vi "SCMP - Write Comments to File.vi"(8 "error in":errorcluster, 9 "data to end":string, 10 "data":string, 11 "Today's SCMP folder":path) -> (0 "error out":errorcluster, 2 "Last Log Entry":string="\r", 3 "Entire Log File":string="\n", 5 "Today's SCMP Log File":path)   [LabVIEW 2014]
doc: "This vi create or open file, which is save in format YYYYMMDD.txt. In this file are logs from CoMP-S Main program."
panel:
  in  "SCMP Log File":path=path "SCMP dump init.log"
  out "first call":bool
  out "date/time string":string="20141030"
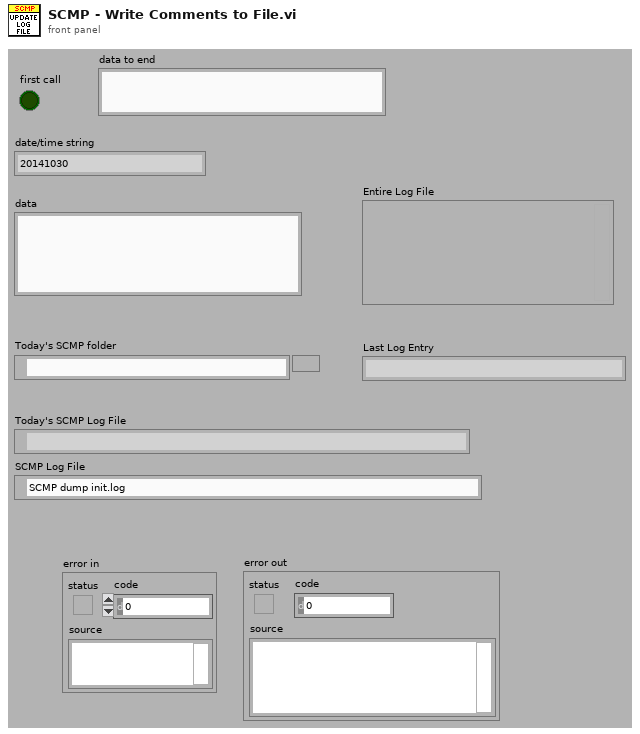
[diagram p1: front panel]
types:
  T1 = enum16{"open", "replace", "create", "open or create", "replace or create", "replace or create with confirmation"}
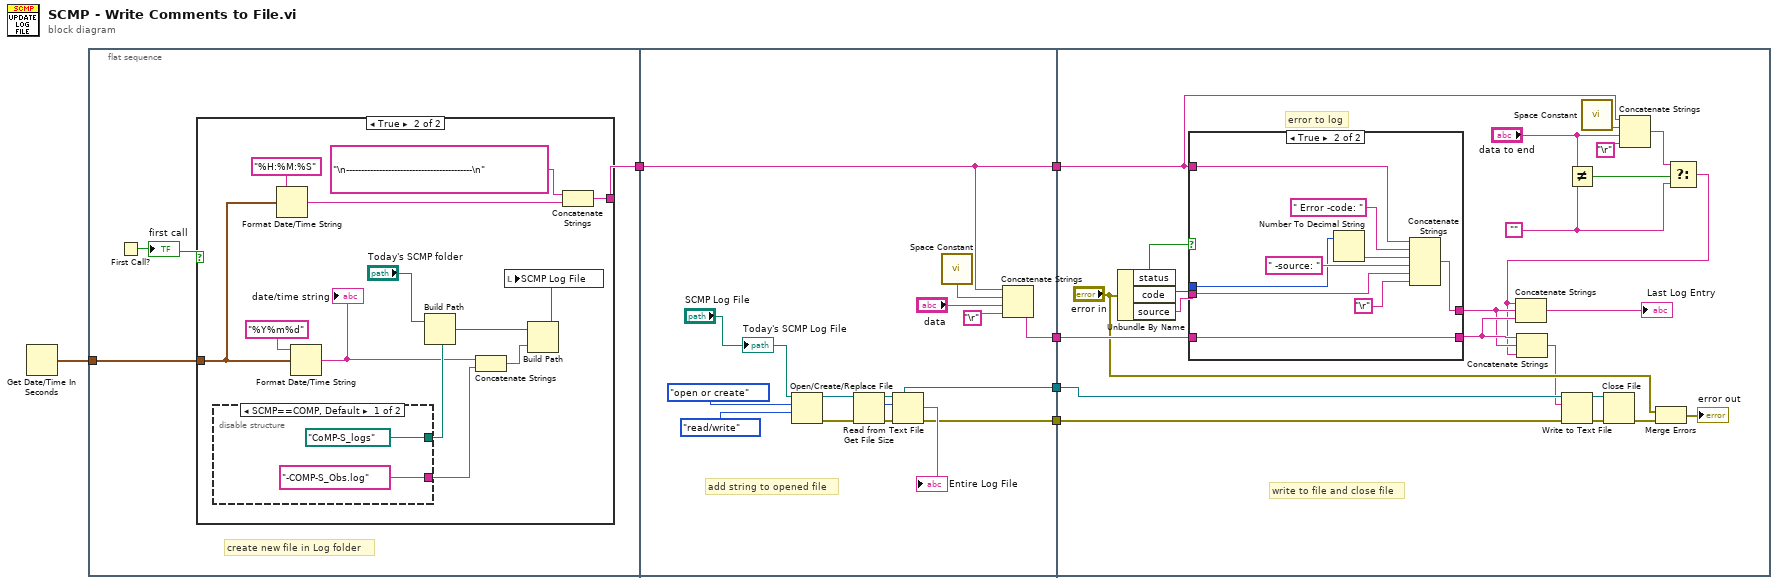
[diagram p0: block diagram]
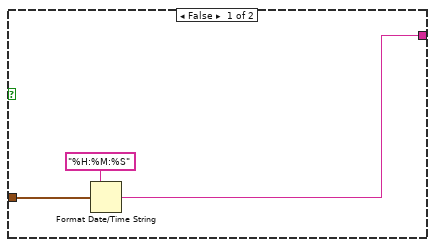
[diagram p2: hidden frame]
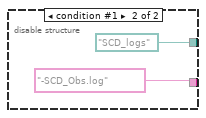
[diagram p3: hidden frame]
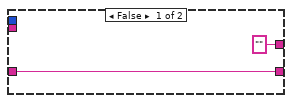
[diagram p4: hidden frame]
diagram:
  n1 = Get Date/Time In Seconds() -> (seconds since 1Jan1904=w3:timestamp)
  n2 = flat-sequence {
    tunnel: w3 -> [w8]
    tunnel: [w7] -> w1
    tunnel: [w34] -> w6
    tunnel: [w35] -> w5
    tunnel: [w30] -> w4
    tunnel: [w32] -> w2
    tunnel: w1 -> [w30]
    tunnel: w6 -> [w62]
    tunnel: w5 -> [w66]
    tunnel: w4 -> [w47]
    tunnel: w2 -> [w61]
    frame #0 {
      # "create new file in Log folder"
      n3 = First Call?() -> (First Call?: T/F=w9:bool)
      "first call" <- w9
      n4 = case shown="True" w9 {
        tunnel: w8 -> [w11 w16]
        tunnel: [w10 w14] -> w7
        frame False {
          n5 = Format Date/Time String(time format string (%c)="%H:%M:%S", seconds (now)=w11) -> (date/time string=w10:string)  [unwired: 1 in]
        }
        frame True {
          n6 = disable-structure shown="SCMP==COMP, Default" {
            disable-tunnel: [path "CoMP-S_logs" path "SCD_logs"] -> w24
            disable-tunnel: ["-COMP-S_Obs.log" ("string") "-SCD_Obs.log" ("string")] -> w20
            frame condition #0 (active) {
            }
            frame condition #1 {
            }
          }
          n7 = Format Date/Time String(time format string (%c)="%H:%M:%S", seconds (now)=w16) -> (date/time string=w13:string)  [unwired: 1 in]
          n8 = Format Date/Time String(time format string (%c)="%Y%m%d", seconds (now)=w16) -> (date/time string=w21:string)  [unwired: 1 in]
          "date/time string" <- w21
          n9 = Build Path(base path="Today's SCMP folder", name or relative path=w24) -> (appended path=w23:path)
          n10 = Concatenate Strings(w21, w20) -> (w22:string)
          n11 = Build Path(base path=w23, name or relative path=w22) -> (appended path=w19:path)
          n12 = local write "SCMP Log File"(w19) -> ()
          n13 = Concatenate Strings("\n------------------------------------------\n" ("date/time string"), w13) -> (w14:string)
        }
      }
    }
    frame #1 {
      # "add string to opened file"
      n14 = Open/Create/Replace File(file path (use dialog)="SCMP Log File", operation (0:open)=T1."open or create", access (0:read/write)=enum16{"read/write", "read-only", "write-only"}."read/write") -> (refnum out=w42:refnum<file>, error out=w41:errorcluster)  [unwired: 1 in, 3 out]
      n15 = Get File Size(file=w42, error in=w41) -> (refnum out=w43:refnum<file>, size (in bytes)=w44:i64, 0:w33:errorcluster)
      n16 = Read from Text File(file (use dialog)=w43, count=w44, error in=w33) -> (refnum out=w35:refnum<file>, text=→"Entire Log File":string, error out=w32:errorcluster)  [unwired: 2 out]
      n17 = call <vilib>:"Space Constant.vi"() -> ("String"=w39:string)
      n18 = Concatenate Strings(w30, w39, "data", "\r") -> (w34:string)
      "Today's SCMP Log File" <- "SCMP Log File"
    }
    frame #2 {
      w50 = ""
      # "error to log"
      # "write to file and close file"
      n19 = Unbundle By Name("error in") -> ("status"=w63:bool, "code"=w64:i32, "source"=w65:string)
      n20 = case shown="True" w63 {
        tunnel: w65 -> [_ w78]
        tunnel: w64 -> [_ w76]
        tunnel: w62 -> [w70 w71]
        tunnel: [w70 w71] -> w57
        tunnel: w47 -> [_ w73]
        tunnel: ["" w72] -> w54
        frame False {
        }
        frame True {
          n21 = Number To Decimal String(number=w76) -> (decimal integer string=w75:string)  [unwired: 1 in]
          n22 = Concatenate Strings(w73, " Error -code: ", w75, " -source: ", w78, "\r") -> (w72:string)
        }
      }
      n23 = Not Equal?(x="data to end", y=w50) -> (x != y?=w51:bool)
      n24 = call <vilib>:"Space Constant.vi"() -> ("String"=w46:string)
      n25 = Concatenate Strings(w47, w46, "data to end", "\r") -> (w49:string)
      n26 = Select(t=w49, s=w51, f=w50) -> (s? t:f=w48:string)
      n27 = Concatenate Strings(w48, w54, w57) -> (→"Last Log Entry":string)
      n28 = Concatenate Strings(w57, w54, w48) -> (w56:string)
      n29 = Write to Text File(file (use dialog)=w66, text=w56, error in=w61) -> (refnum out=w67:refnum<file>, error out=w68:errorcluster)  [unwired: 1 in, 1 out]
      n30 = Close File(refnum=w67, error in=w68) -> (error out=w59:errorcluster)  [unwired: 1 out]
      n31 = Merge Errors("error in", w59) -> (→"error out":errorcluster)
    }
  }
